vi "SetStatusRatesSparkMax.vi"(11 "MotorControlDeviceRef In":T2={"DeviceStatus"={"status"=FALSE, "code"=0, "source"=""}, "Type"=enum."PWM", "PWM"={"PWM Channel"=enum."Invalid", "DeadBand"={"Name"="", "maxPositivePwm"=0, "minPositivePwm"=0, "centerPwm"=0, "maxNegativePwm"=0, "minNegativePwm"=0, "angularRange"=0}}, "CAN"={"Device Number"=0, "SetOutput VI Ref"=variant(refnum<vi> refnum), "GetOutput VI Ref"=variant(refnum<vi> refnum), "Enable VI Ref"=variant(refnum<vi> refnum), "Disable VI Ref"=variant(refnum<vi> refnum), "Data"=variant}, "Invert"=FALSE, "DIO PWM"={"PWM \"Enable\" Channel"=enum."Invalid", "DIOChannel"=enum."Invalid", "PWM Rate"=0.0}}) -> (3 "MotorControlDeviceRef Out":T2={"DeviceStatus"={"status"=FALSE, "code"=0, "source"=""}, "Type"=enum."PWM", "PWM"={"PWM Channel"=enum."Invalid", "DeadBand"={"Name"="", "maxPositivePwm"=0, "minPositivePwm"=0, "centerPwm"=0, "maxNegativePwm"=0, "minNegativePwm"=0, "angularRange"=0}}, "CAN"={"Device Number"=0, "SetOutput VI Ref"=variant(refnum<vi> refnum), "GetOutput VI Ref"=variant(refnum<vi> refnum), "Enable VI Ref"=variant(refnum<vi> refnum), "Disable VI Ref"=variant(refnum<vi> refnum), "Data"=variant}, "Invert"=FALSE, "DIO PWM"={"PWM \"Enable\" Channel"=enum."Invalid", "DIOChannel"=enum."Invalid", "PWM Rate"=0.0}})   [LabVIEW 2018]
uses:
  <vilib>/Rock Robotics/WPI/MotorControl/WPI_MotorControlDeviceRef.ctl
  <vilib>/Rock Robotics/WPI/MotorControl/WPI_MotorControlType.ctl
  <vilib>/Rock Robotics/SystemInterfaces/DIO/FPGA_DIOPWMChannel.ctl
  <vilib>/Rock Robotics/WPI/PWM/WPI_PWMDeadband.ctl
  <vilib>/Rock Robotics/SystemInterfaces/DIO/FPGA_DIOChannel.ctl
  <vilib>/Rock Robotics/WPI/ThirdParty/REV Robotics/SPARK MAX/Typedef/Spark MAX Status Frames.ctl
panel:
  in  "StatusRates":T1={"Status 0 (ms)"=65535, "Status 1 (ms)"=20, "Status 2 (ms)"=20, "Status 3 (ms)"=65535}
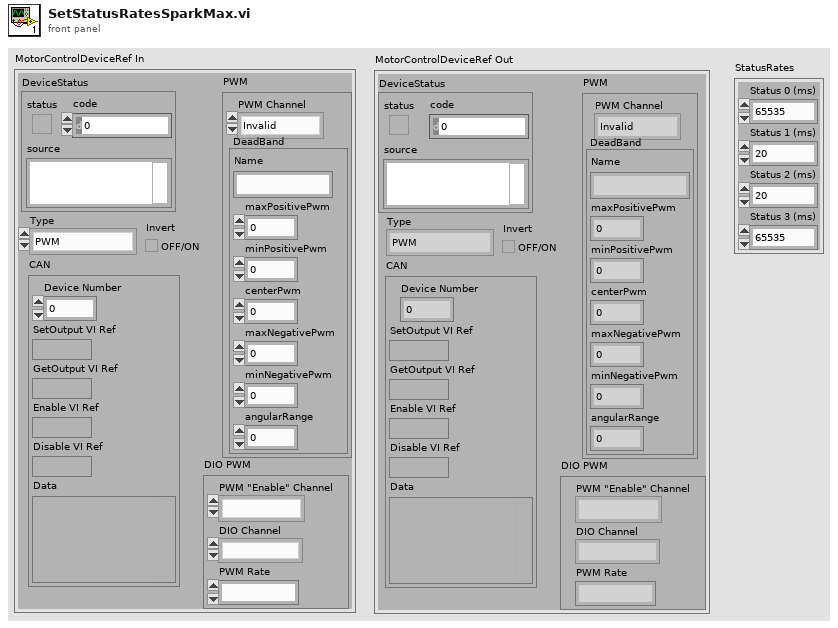
[diagram p1: front panel]
types:
  T1 = cluster{"Status 0 (ms)":u16, "Status 1 (ms)":u16, "Status 2 (ms)":u16, "Status 3 (ms)":u16}
  T2 = typedef "WPI_MotorControlDeviceRef.ctl" = cluster{"DeviceStatus":errorcluster, "Type":T3, "PWM":cluster{"PWM Channel":T4, "DeadBand":T5}, "CAN":cluster{"Device Number":u8, "SetOutput VI Ref":variant, "GetOutput VI Ref":variant, "Enable VI Ref":variant, "Disable VI Ref":variant, "Data":variant}, "Invert":bool, "DIO PWM":cluster{"PWM \"Enable\" Channel":T4, "DIOChannel":T6, "PWM Rate":dbl}}
  T3 = typedef "WPI_MotorControlType.ctl" = enum16{"PWM", "CAN", "DIO PWM"}
  T4 = typedef "FPGA_DIOPWMChannel.ctl" = enum8{"PWM 0", "PWM 1", "PWM 2", "PWM 3", "PWM 4", "PWM 5", "PWM 6", "PWM 7", "PWM 8", "PWM 9", "PWM MXP 0", "PWM MXP 1", "PWM MXP 2", "PWM MXP 3", "PWM MXP 4", "PWM MXP 5", "PWM MXP 6", "PWM MXP 7", "PWM MXP 8", "PWM MXP 9", "Invalid"}
  T5 = typedef "WPI_PWMDeadband.ctl" = cluster{"Name":string, "maxPositivePwm":i32, "minPositivePwm":i32, "centerPwm":i32, "maxNegativePwm":i32, "minNegativePwm":i32, "angularRange":u16}
  T6 = typedef "FPGA_DIOChannel.ctl" = enum8{"DIO 0", "DIO 1", "DIO 2", "DIO 3", "DIO 4", "DIO 5", "DIO 6", "DIO 7", "DIO 8", "DIO 9", "DIO MXP 0", "DIO MXP 1", "DIO MXP 2", "DIO MXP 3", "DIO MXP 4", "DIO MXP 5", "DIO MXP 6", "DIO MXP 7", "DIO MXP 8", "DIO MXP 9", "DIO MXP 10", "DIO MXP 11", "DIO MXP 12", "DIO MXP 13", "DIO MXP 14", "DIO MXP 15", "SPI Port CS1", "SPI Port CS2", "SPI Port CS3", "SPI Port MISO", "SPI Port MOSI", "Invalid"}
  T7 = typedef "Spark MAX Status Frames.ctl" = enum16{"Status 0", "Status 1", "Status 2", "Status 3"}
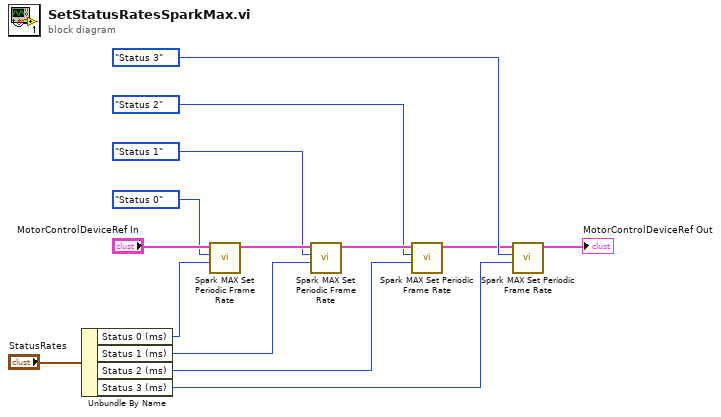
[diagram p0: block diagram]
diagram:
  n1 = Unbundle By Name("StatusRates") -> ("Status 0 (ms)"=w4:u16, "Status 1 (ms)"=w3:u16, "Status 2 (ms)"=w2:u16, "Status 3 (ms)"=w1:u16)
  n2 = call <vilib>:"Spark MAX Set Periodic Frame Rate.vi"("Frame rate (ms)"=w4, "Frame"=Spark_MAX_Status_Frames."Status 0", "MotorControlDeviceRef"="MotorControlDeviceRef In") -> ("MotorControlDeviceRef"=w12:T2)  [unwired: 7 in, 1 out]
  n3 = call <vilib>:"Spark MAX Set Periodic Frame Rate.vi"("Frame rate (ms)"=w3, "Frame"=Spark_MAX_Status_Frames."Status 1", "MotorControlDeviceRef"=w12) -> ("MotorControlDeviceRef"=w11:T2)  [unwired: 7 in, 1 out]
  n4 = call <vilib>:"Spark MAX Set Periodic Frame Rate.vi"("Frame rate (ms)"=w2, "Frame"=Spark_MAX_Status_Frames."Status 2", "MotorControlDeviceRef"=w11) -> ("MotorControlDeviceRef"=w7:T2)  [unwired: 7 in, 1 out]
  n5 = call <vilib>:"Spark MAX Set Periodic Frame Rate.vi"("Frame rate (ms)"=w1, "Frame"=Spark_MAX_Status_Frames."Status 3", "MotorControlDeviceRef"=w7) -> ("MotorControlDeviceRef"=→"MotorControlDeviceRef Out":T2)  [unwired: 7 in, 1 out]
